vi "Stop Core.vi"(10 "final error code":i32, 11 "MFC in":refnum<class "Control.lvclass">) -> (3 "MFC out":refnum<class "Control.lvclass">)   [LabVIEW 2013, in "Control.lvib.lvlib" / "Control.lvclass"]
doc: "(<B>Filename</B>: Actor Framework.lvlib:Actor.lvclass:Stop Core.vi)\n\nDefines what the actor does before it stops. Use the <B>final error code</B> input to determine whether the actor shut down in response to an error.\n\nBy default, this method does nothing. A descendant class may override it to define behavior, such as shutting down any processes the actor initiated in its override of the Actor Core method."
uses:
  Control.lvclass
  PluginInterface/PluginInterface.lvlibp/PluginInterfaceClass/PluginInterface.lvclass
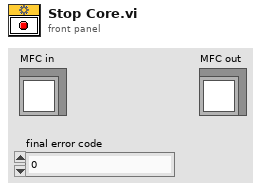
[diagram p1: front panel]
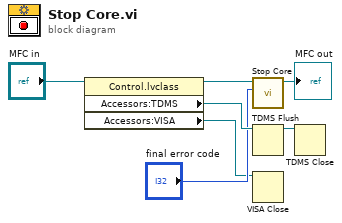
[diagram p0: block diagram]
diagram:
  n1 = property class="Control.lvclass"(reference="MFC in") -> (reference out=w7:refnum<class "Control.lvclass">, "Accessors:TDMS"=w6:refnum<k34>, "Accessors:VISA"=w1:refnum<visa-resource-name>)  [unwired: 1 in, 1 out]
  n2 = call-parent "Stop Core.vi"("final error code"="final error code", "Actor in"=w7) -> ("Actor out"=→"MFC out":refnum<class "Control.lvclass">)  [unwired: 9 in]
  n3 = TDMS Flush(7:w6) -> (3:w2:refnum<k34>)  [unwired: 1 in, 1 out]
  n4 = VISA Close(VISA resource name=w1) -> ()  [unwired: 1 in, 1 out]
  n5 = TDMS Close(11:w2) -> ()  [unwired: 1 in, 2 out]
